vi "constants.vi"() -> ()   [LabVIEW 2019]
doc: "These global variables store constant values configured in Begin."
panel:
  out "Legal_MVP_Overrides":string[](array[string])
  out "Legal_Actuator_Names":string[](array[string])
  out "Possible_Shooter_States":string[](array[string])
  out "Possible_States":string[](array[string])
  out "Legal_Auto_Plays":string[](array[string])
  out "Legal_Drivers":string[](array[string])
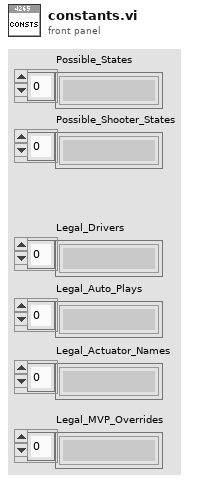
[diagram p1: front panel]
diagram:
